vi "PCO_SetROI.vi"(0 "ph":u64, 1 "wRoiX0":u16, 2 "wRoiX1":u16, 11 "error in (no error)":errorcluster {"code" format="%x"}, 12 "wRoiY0":u16, 13 "wRoiY1":u16) -> (4 "ph out":u64, 6 "ErrorMessage":i32 format="%x", 15 "error out":errorcluster {"code" format="%x"})   [LabVIEW 2020, in "SDK.lvlib" / "ImageSensor.lvlib"]
doc: "<b>Description:</b>\nThis function does set a ROI (region of interest) area on the sensor of the camera.\nSee chapter IMAGE AREA SELECTION (ROI) how valid input parameters can be determined.\nInvalid values will result in a failure response message either immediately or from next PCO_ArmCamera call.\nThe command will be rejected, if Recording State is [run], see PCO_GetRecordingState.\n\n<b>Supported camera type:</b>\npco.edge, pco.dimax, pco.1200, pco.1600, pco.2000, pco.4000\n\n<b>Descriptor dependency:</b>\nwRoiHorStepsDESC, wRoiVertStepsDESC"
uses:
  ImageSensor.lvlib
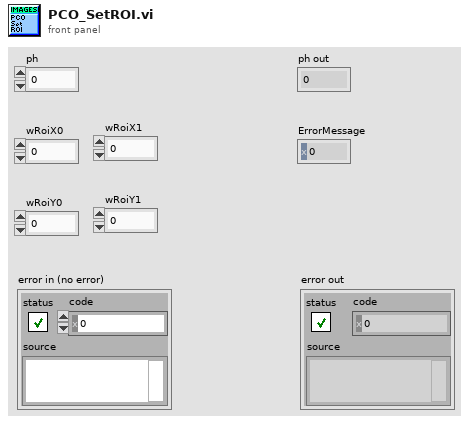
[diagram p1: front panel]
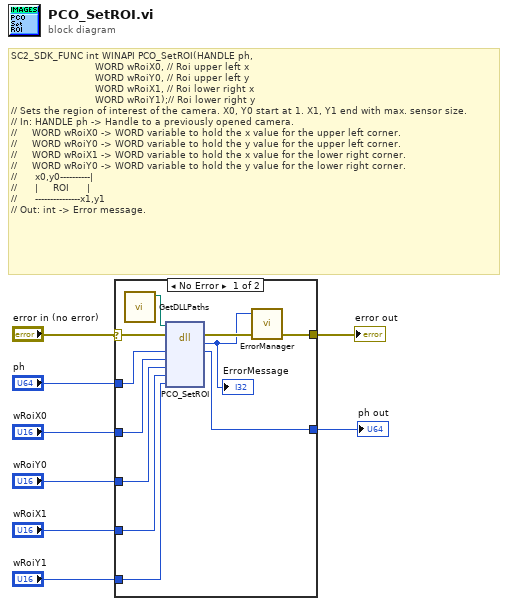
[diagram p0: block diagram]
diagram:
  # "SC2_SDK_FUNC int WINAPI PCO_SetROI(HANDLE ph,\n                            WORD wRoiX0, // Roi upper left x\n                            WORD wRoiY0, // Roi upper left y\n                            WORD wRoiX1, // Roi lower right x\n                            WORD wRoiY1);// Roi lower right y\n// Sets the region of interest of the camera. X0, Y0 start at 1. X1, Y1 end with max. sensor size.\n// In: HANDLE ph -> Handle to a previously opened camera.\n//     WORD wRoiX0 -> WORD variable to hold the x value for the upper left corner.\n//     WORD wRoiY0 -> WORD variable to hold the y value for the upper left corner.\n//     WORD wRoiX1 -> WORD variable to hold the x value for the lower right corner.\n//     WORD wRoiY0 -> WORD variable to hold the y value for the lower right corner.\n//      x0,y0----------|\n//      |     ROI      |\n//      ---------------x1,y1\n// Out: int -> Error message."
  n1 = case shown="No Error" "error in (no error)" {
    selector: "error in (no error)" -> [w13 w21]
    tunnel: "ph" -> [w19 w20]
    tunnel: [w18 w20] -> w7
    tunnel: "wRoiX0" -> [w17 _]
    tunnel: "wRoiY0" -> [w16 _]
    tunnel: "wRoiX1" -> [w15 _]
    tunnel: "wRoiY1" -> [w14 _]
    tunnel: [w11 w21] -> w2
    frame No Error {
      n2 = call "GetDLLPaths.vi"() -> ("SC2_Cam_Path"=w9:path)  [unwired: 9 in, 2 out]
      n3 = dll-call lib="?" fn="PCO_SetROI"(path in=w9, error in=w13, "ph"=w19, "wRoiX0"=w17, "wRoiY0"=w16, "wRoiX1"=w15, "wRoiY1"=w14) -> (error out=w12:errorcluster, "return type"=w10:i32, "ph"=w18:u64)  [unwired: 5 in, 1 out]
      "ErrorMessage" <- w10
      n4 = call "ErrorManager.vi"("error in (no error)"=w12, "error code"=w10) -> ("error out"=w11:errorcluster)  [unwired: 3 in]
    }
    frame Error {
    }
  }
  "ph out" <- w7
  "error out" <- w2
